vi "Get_Intensity_Value_For_Thresholding-2.vi"(4 "[IN] Index for \nthresholding":i8, 5 "error IN":errorcluster, 6 "[IN] Binarization Set\ntings (Both Channels)":cluster{"MinBin2":sgl, "MaxBin2":sgl}[](array[cluster]), 7 "[IN] 1 or 2 channel":u8, 8 "[IN] Index of starting \npoint for thresholding":i32) -> (0 "error OUT":errorcluster, 1 "[OUT] Binarization Set\ntings (Both Channels)":cluster{"MinBin2":sgl, "MaxBin2":sgl}[](array[cluster]), 2 "[OUT] For Operator \nBinarization Values":cluster{"MinBin2":sgl, "MaxBin2":sgl})   [LabVIEW 2013]
doc: "SubVI saves used for thresholding limits (255 - commonly highest value, user defines only 1 value for threshold)"
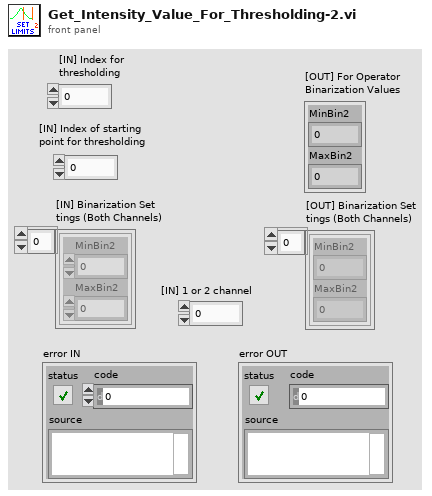
[diagram p1: front panel]
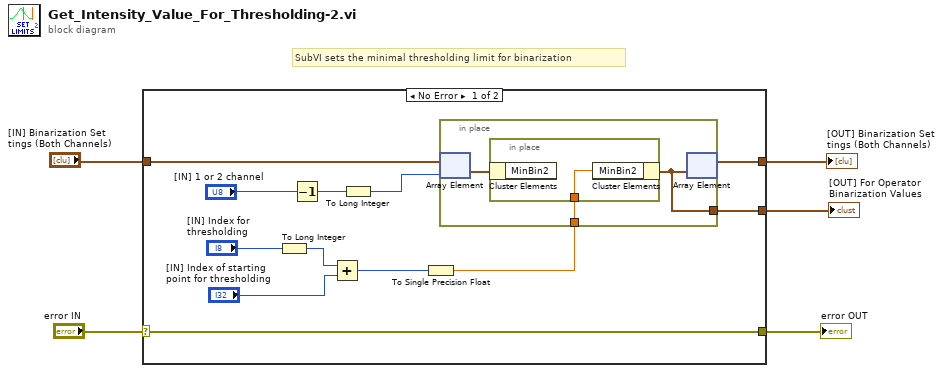
[diagram p0: block diagram]
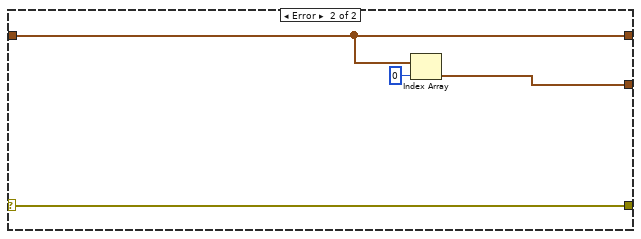
[diagram p2: hidden frame]
diagram:
  # "SubVI sets the minimal thresholding limit for binarization"
  n1 = case shown="No Error" "error IN" {
    selector: "error IN" -> [w13 w25]
    tunnel: [w13 w25] -> w4
    tunnel: [w8 w24] -> w2
    tunnel: "[IN] Binarization Set\ntings (Both Channels)" -> [w7 w24]
    tunnel: [w6 w22] -> w1
    frame No Error {
      n2 = To Long Integer(number="[IN] Index for \nthresholding") -> (32bit integer=w16:i32)
      n3 = Decrement(x="[IN] 1 or 2 channel") -> (x-1=w11:u8)
      n4 = Add(x=w16, y="[IN] Index of starting \npoint for thresholding") -> (x+y=w17:i32)
      n5 = To Long Integer(number=w11) -> (32bit integer=w10:i32)
      n6 = To Single Precision Float(number=w17) -> (single precision float=w9:sgl)
      n7 = in-place {
        in-place-border: w9 -> [w19]
        in-place-border: [w18] -> w6
        n8 = in-place-array #1(w7, w10) -> (w20:cluster{"MinBin2":sgl, "MaxBin2":sgl})
        n9 = in-place {
          in-place-border: w19 -> [w21]
          n10 = in-place-cluster #2(w20) -> ()  [unwired: 1 out]
          n11 = in-place-cluster #2("MinBin2"=w21) -> (w18:cluster{"MinBin2":sgl, "MaxBin2":sgl})
        }
        n12 = in-place-array #1(w18) -> (w8:cluster{"MinBin2":sgl, "MaxBin2":sgl}[])  [unwired: 1 out]
      }
    }
    frame Error {
      n13 = Index Array(array=w24, index=0) -> (element=w22:cluster{"MinBin2":sgl, "MaxBin2":sgl})
    }
  }
  "error OUT" <- w4
  "[OUT] Binarization Set\ntings (Both Channels)" <- w2
  "[OUT] For Operator \nBinarization Values" <- w1
